vi "Read SN.vi"(8 "error in (no error)":errorcluster, 11 "PPT in":refnum<class "PPT.lvclass">) -> (0 "error out":errorcluster, 2 "SN":string caption="Address", 3 "PPT out":refnum<class "PPT.lvclass">)   [LabVIEW 2014, in "PPT Library.lvlib" / "PPT.lvclass"]
uses:
  PPT.lvclass
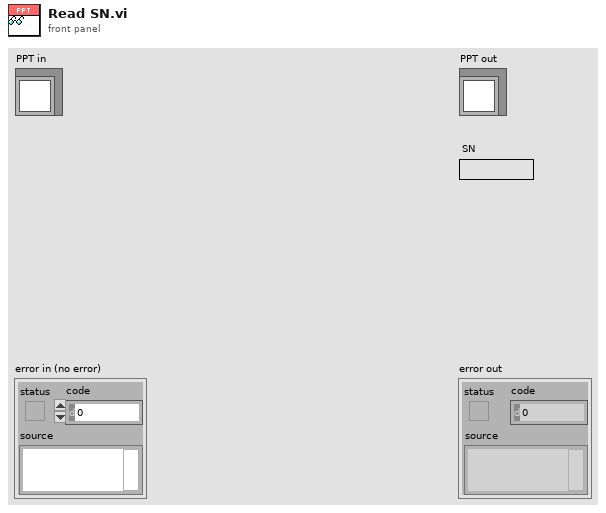
[diagram p1: front panel]
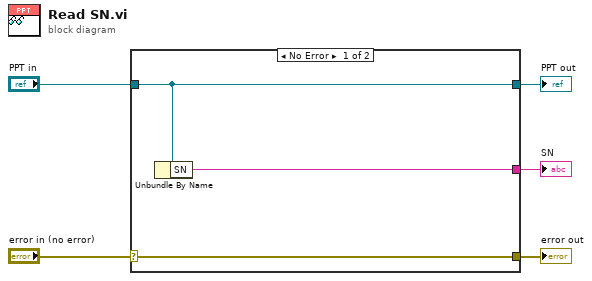
[diagram p0: block diagram]
diagram:
  n1 = case shown="No Error" "error in (no error)" {
    selector: "error in (no error)" -> [w8 w9]
    tunnel: [w8 w9] -> w4
    tunnel: [w7 w10] -> w2
    tunnel: "PPT in" -> [w7 w10]
    tunnel: [w6 _] -> w1
    frame No Error {
      n2 = Unbundle By Name(w7) -> ("SN"=w6:string)
    }
    frame Error {
    }
  }
  "error out" <- w4
  "PPT out" <- w2
  "SN" <- w1
